vi "Receive.vi"(11 "jettl in":refnum<class "jettl.lvclass">) -> (2 "Msg":refnum<class "Msg.lvclass">, 3 "jettl out":refnum<class "jettl.lvclass">)   [LabVIEW 2021, in "jettl.lvlib" / "jettl.lvclass"]
uses:
  jettl.lvclass
  Actor/Msg/Msg.lvclass
  jettl.lvclass/jettl.ctl
  State/State/State.lvclass
  jettl.lvlib
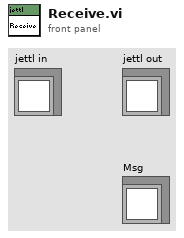
[diagram p1: front panel]
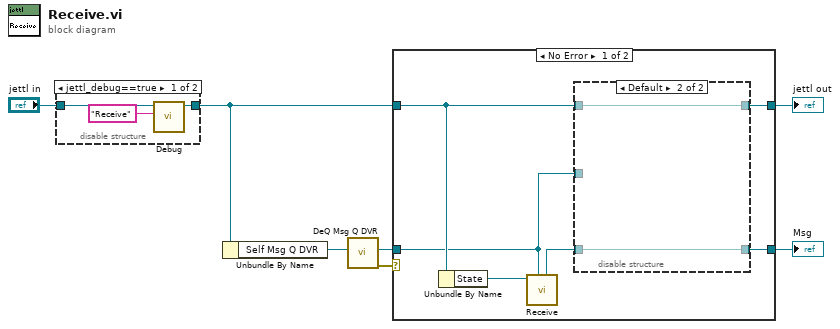
[diagram p0: block diagram]
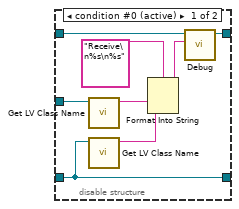
[diagram p3: hidden frame]
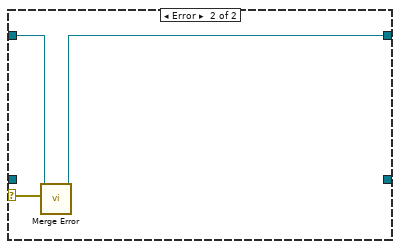
[diagram p4: hidden frame]
diagram:
  n1 = disable-structure shown="jettl_debug==true" {
    disable-tunnel: "jettl in" -> [w10 w11]
    disable-tunnel: [w9 w11] -> w3
    frame condition #0 (active) {
      n2 = call "Debug.vi"("Method"="Receive", "jettl in"=w10) -> ("jettl out"=w9:refnum<class "jettl.lvclass">)  [unwired: 9 in]
    }
    frame condition #1 {
    }
  }
  n3 = Unbundle By Name(w3) -> ("Self Msg Q DVR"=w7:refnum<data-value>)
  n4 = call "DeQ Msg Q DVR.vi"("Msg Q DVR"=w7) -> ("error out"=w6:errorcluster, "Msg"=w5:refnum<class "Msg.lvclass">)  [unwired: 9 in]
  n5 = case shown="No Error" w6 {
    selector: w6 -> [_ w28]
    tunnel: [w13 _] -> w2
    tunnel: w5 -> [w12 _]
    tunnel: w3 -> [w16 w30]
    tunnel: [w15 w29] -> w1
    frame No Error {
      n6 = Unbundle By Name(w16) -> ("State"=w17:refnum<class "State.lvclass">)
      n7 = call-dynamic "Receive.vi"("Msg in"=w12, "State in"=w17) -> ("Msg out"=w14:refnum<class "Msg.lvclass">)  [unwired: 9 in]
      n8 = disable-structure shown="Default" {
        disable-tunnel: w16 -> [w25 w27]
        disable-tunnel: [w24 w27] -> w15
        disable-tunnel: [w23 w26] -> w13
        disable-tunnel: w14 -> [w23 w26]
        disable-tunnel: w12 -> [w22 _]
        frame condition #0 (active) {
          n9 = call <vilib>:"Get LV Class Name.vi"("object"=w22) -> ("class name"=w21:string)  [unwired: 9 in, 1 out]
          n10 = call <vilib>:"Get LV Class Name.vi"("object"=w23) -> ("class name"=w19:string)  [unwired: 9 in, 1 out]
          n11 = Format Into String(format string="Receive\n%s\n%s" ("Method"), w21, w19) -> (resulting string=w18:string)  [unwired: 2 in, 1 out]
          n12 = call "Debug.vi"("Method"=w18, "jettl in"=w25) -> ("jettl out"=w24:refnum<class "jettl.lvclass">)  [unwired: 9 in]
        }
        frame condition #1 {
        }
      }
    }
    frame Error {
      n13 = call-dynamic "Merge Error.vi"("Error"=w28, "jettl in"=w30) -> ("jettl out"=w29:refnum<class "jettl.lvclass">)  [unwired: 9 in]
    }
  }
  "Msg" <- w2
  "jettl out" <- w1
